vi "Control_PP_Blocks.vi"() -> (5 "Plug in titles":string[](array[string]), 7 "Plug in values":string[](array[string]))   [LabVIEW 2016]
uses:
  Globals/Meas_global.vi
  Post_Processing_specials/Block_Control_global.vi
panel:
  in  "No of Blocks to PP":i32=1 min=1
  in  "Start Block Number":i32=1 min=1
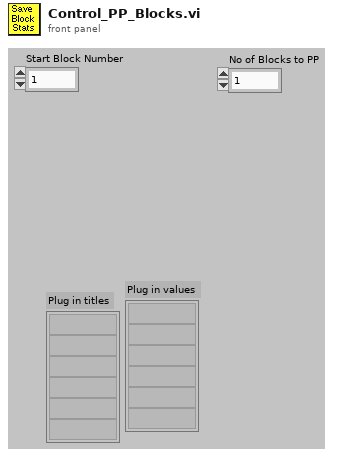
[diagram p1: front panel]
types:
  T1 = typedef "Post_Process.ctl" = enum16{"Take New Data", "Post Process Raw Data File"}
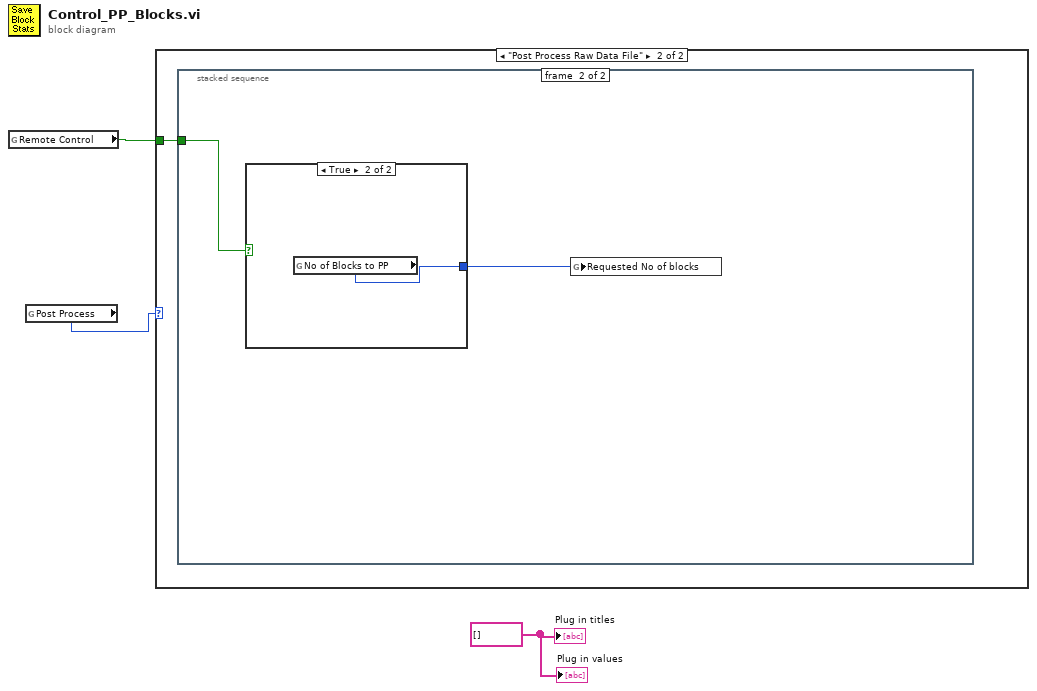
[diagram p0: block diagram]
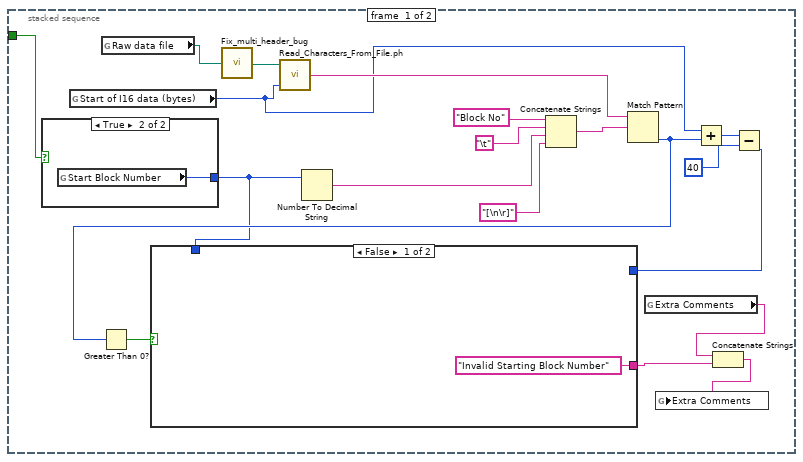
[diagram p3: hidden frame]
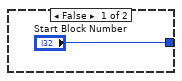
[diagram p4: hidden frame]
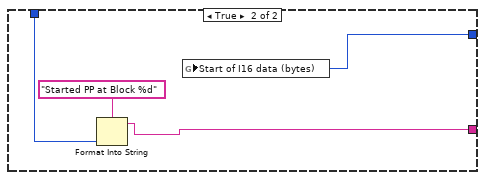
[diagram p5: hidden frame]
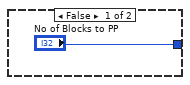
[diagram p6: hidden frame]
diagram:
  w2 = string[] [] ("Plug in titles")
  n1 = global read "Block_Control_global.vi" "Remote Control"() -> (w1:bool)
  n2 = global read "Meas_global.vi" "Post Process"() -> (w3:T1)
  n3 = case shown="\"Post Process Raw Data File\"" w3 {
    tunnel: w1 -> [_ w4]
    frame "Take New Data" {
    }
    frame "Post Process Raw Data File" {
      n4 = stacked-sequence {
        tunnel: w4 -> [w9 w31]
        frame #0 {
          n5 = case shown="True" w9 {
            tunnel: ["Start Block Number" w25] -> w8
            frame False {
            }
            frame True {
              n6 = global read "Block_Control_global.vi" "Start Block Number"() -> (w25:i32)
            }
          }
          n7 = global read "Meas_global.vi" "Start of I16 data (bytes)"() -> (w15:i32)
          n8 = global read "Meas_global.vi" "Raw data file"() -> (w23:path)
          n9 = call "Fix_multi_header_bug.vi"("Raw data File to Read"=w23) -> ("Raw data File to Read Out"=w22:path)
          n10 = call "Read_Characters_From_File.ph.vi"("file path (dialog if empty)"=w22, "start of read offset (chars.: 0)"=w15) -> ("character string"=w17:string)  [unwired: 4 in, 3 out]
          n11 = Number To Decimal String(number=w8) -> (decimal integer string=w19:string)  [unwired: 1 in]
          n12 = Concatenate Strings("Block No", "\t", w19, "[\n\r]") -> (w18:string)
          n13 = Match Pattern(string=w17, regular expression=w18) -> (offset past match=w12:i32)  [unwired: 1 in, 3 out]
          n14 = Greater Than 0?(x=w12) -> (x > 0?=w11:bool)
          n15 = global read "Meas_global.vi" "Extra Comments"() -> (w7:string)
          n16 = Add(x=w15, y=w12) -> (x+y=w14:i32)
          n17 = Subtract(x=w14, y=40) -> (x-y=w10:i32)
          n18 = case shown="False" w11 {
            tunnel: w10 -> [_ w29]
            tunnel: w8 -> [_ w28]
            tunnel: ["Invalid Starting Block Number" w27] -> w6
            frame False {
            }
            frame True {
              n19 = Format Into String(format string="Started PP at Block %d", w28) -> (resulting string=w27:string)  [unwired: 2 in, 1 out]
              n20 = global write "Meas_global.vi" "Start of I16 data (bytes)"(w29) -> ()
            }
          }
          n21 = Concatenate Strings(w7, w6) -> (w5:string)
          n22 = global write "Meas_global.vi" "Extra Comments"(w5) -> ()
        }
        frame #1 {
          n23 = case shown="True" w31 {
            tunnel: ["No of Blocks to PP" w34] -> w32
            frame False {
            }
            frame True {
              n24 = global read "Block_Control_global.vi" "No of Blocks to PP"() -> (w34:i32)
            }
          }
          n25 = global write "Meas_global.vi" "Requested No of blocks"(w32) -> ()
        }
      }
    }
  }
  "Plug in values" <- w2
  "Plug in titles" <- w2
